vi "ConvertPayloadToPayloadStr.vi"(11 "payload":u8[](array[numeric]) format="%x") -> (3 "string-hex":string)   [LabVIEW 2018, in "Library-DataConvert.lvlib"]
uses:
  Library-DataConvert.lvlib
  <vilib>/Utility/error.llb/whitespace.ctl
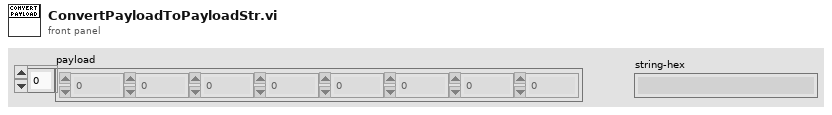
[diagram p1: front panel]
types:
  T1 = typedef "whitespace.ctl" = u16
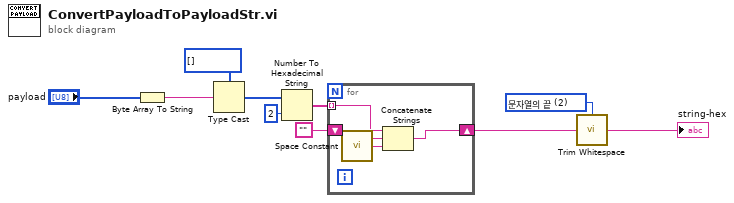
[diagram p0: block diagram]
diagram:
  w5 = T1 2 items=["모두", "문자열의 시작", "문자열의 끝"] ("location (both)")
  n1 = Byte Array To String(unsigned byte array="payload") -> (string=w1:string)
  n2 = Type Cast(type=i8[] [], x=w1) -> (*(type *) &x=w6:i8[])
  n3 = Number To Hexadecimal String(1:i16 2 ("폭(-)"), 2:w6) -> (0:w10:string[])
  n4 = for {
    tunnel: w10 -> [w12] mode=indexing
    shift-right: [w14] -> w4
    shift-left: "" -> [w13]
    n5 = call <vilib>:"Space Constant.vi"() -> ("String"=w11:string)
    n6 = Concatenate Strings(w13, w12, w11) -> (w14:string)
  }
  n7 = call <vilib>:"Trim Whitespace.vi"("string"=w4, "location (both)"=w5) -> ("trimmed string"=→"string-hex":string)
